vi "Position Based Vacuum Force.vi"(8 "vac_bnd":dbl[](array[numeric])=[80.0, 100.0], 9 "z_thld":dbl[](array[numeric])=[0.5, 2.5], 10 "current zp":dbl, 11 "tip position":dbl[](array[numeric])) -> (3 "vacf (%)":dbl)   [LabVIEW 2016]
doc: "This VI calculates the vacuum force based on the distance to posterior capsule.\nDistance to posterior capsule is calculated by (current z) - (current zp)\nThe vacuum force is scheduled with some threshold values:\nif z_dist < z_thld(0), vacf = vac_bnd(0);\nif z_dist > z_thld(1), vacf = vac_bnd(1);\nif z_dist is somewhere in between, it propagates linearly."
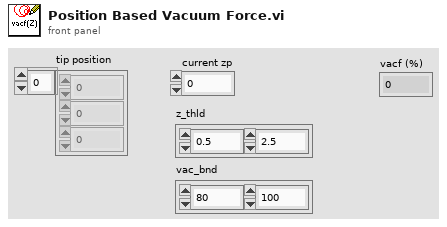
[diagram p1: front panel]
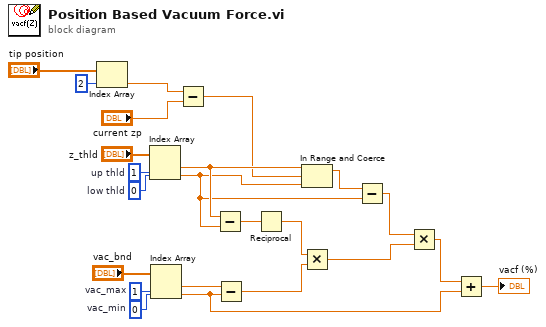
[diagram p0: block diagram]
diagram:
  w18 = 0  # vac_min
  w19 = 1  # vac_max
  w21 = 0  # low thld
  w22 = 1  # up thld
  n1 = Index Array(array="tip position", index=2) -> (element=w1:dbl)
  n2 = Index Array(array="z_thld", index #1=w22, index #2=w21) -> (element #1=w17:dbl, element #2=w11:dbl)
  n3 = Index Array(array="vac_bnd", index #1=w19, index #2=w18) -> (element #1=w16:dbl, element #2=w10:dbl)
  n4 = Subtract(x=w1, y="current zp") -> (x-y=w4:dbl)
  n5 = Subtract(x=w17, y=w11) -> (x-y=w15:dbl)
  n6 = Subtract(x=w16, y=w10) -> (x-y=w13:dbl)
  n7 = Reciprocal(x=w15) -> (1/x=w14:dbl)
  n8 = In Range and Coerce(upper limit=w17, x=w4, lower limit=w11) -> (coerced(x)=w12:dbl)  [unwired: 1 out]
  n9 = Multiply(x=w14, y=w13) -> (x*y=w8:dbl)
  n10 = Subtract(x=w12, y=w11) -> (x-y=w9:dbl)
  n11 = Multiply(x=w9, y=w8) -> (x*y=w7:dbl)
  n12 = Add(x=w7, y=w10) -> (x+y=→"vacf (%)":dbl)
